vi "Read Power Impl.vi"(8 "error in (no error)":errorcluster, 11 "Power Meter in":refnum<class "Power Meter.lvclass">) -> (0 "error out":errorcluster, 2 "Raw Device Reading (W)":dbl=-1.0 caption="Power", 3 "Power Meter out":refnum<class "Power Meter.lvclass">)   [LabVIEW 2023, in "Power Meter.lvlib" / "Power Meter.lvclass"]
uses:
  Power Meter.lvclass
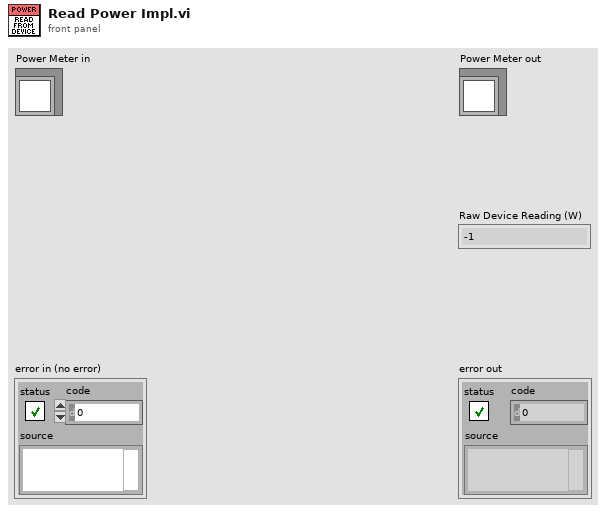
[diagram p1: front panel]
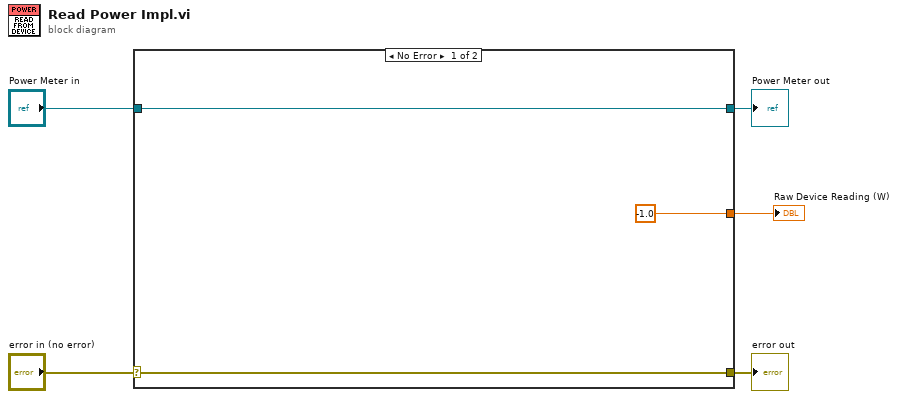
[diagram p0: block diagram]
diagram:
  n1 = case shown="No Error" "error in (no error)" {
    selector: "error in (no error)" -> [w7 w10]
    tunnel: [w7 w10] -> w4
    tunnel: [w8 w9] -> w2
    tunnel: "Power Meter in" -> [w8 w9]
    tunnel: [-1.0 ("Raw Device Reading (W)") _] -> w1
    frame No Error {
    }
    frame Error {
    }
  }
  "error out" <- w4
  "Power Meter out" <- w2
  "Raw Device Reading (W)" <- w1
